vi "comet_thermo_parse_value_html.vi"(8 "error in":errorcluster, 11 "String":string="<!DOCTYPE HTML PUBLIC \"-//W3C//DTD HTML 4.01 Transitional//EN\">\n<html>\n<head>\n <meta http-equiv=\"refresh\" content=\"60\">\n <meta http-equiv=\"content-type\" content=\"text/html; charset=windows-1250\">\n <title>Device: lab7004_JVS</title>\n <style type=\"text/css\">\n <!--\n  h1 {font-size: 1.6em;\tfont-weight: normal;}  \n  .tb {padding:10px 0 0 10px; margin:20px 10px 0 0; height:89px; background:#dee; border:1px solid #000; position:relative;}\n  .ts {padding:0 0 0 0; margin:0 0 0 0; list-style:none; }\n  .ts li {float:left; margin-right:-4px; margin-bottom:-1px;}\n  .ts li a {display:block; text-decoration:none; font-size:11px; font-family:verdana, arial, sans-serif; line-height:23px;}\n  .ts li a em {display:block; float:left; height:25px;text-align:center; padding:0 15px; background:#488; border:1px solid #000; border-right:0; font-style:normal; color:#fff;}\n  .ts li a span {display:none;}\n  .ts li a b {position:relative; display:block; float:left; z-index:100; border-bottom:1px solid #000; width:2px; background:url(tab.gif);}\n  .ts li a b.p1 {height:25px; margin-top:1px;}\n  .ts li a b.p2 {height:23px; margin-top:3px;}\n  .ts li a b.p3 {height:21px; margin-top:5px;}\n  .ts li a b.p4 {height:19px; margin-top:7px;}\n  .ts li a b.p5 {height:18px; width:1px; background:#000; margin-top:9px; font-size:1px; line-height:0; border:0;}\n  .ts li a:hover {color:#000; white-space:normal;}\n  .ts li a:hover em {background:#9bb; color:#000; cursor:pointer; border-bottom-color:#9bb; position:relative; z-index:300;}\n  .ts li a.selected em {background:#9bb; color:#000; border-bottom-color:#9bb; text-decoration:underline; position:relative; z-index:400;}\n  .ts li a.selected:hover em {cursor:default;}\n  .ts li a.selected:hover b {cursor:default;}\n  .ts li a.selected b {z-index:400; background-position:0 -33px; border-bottom-color:#9bb; cursor:pointer;}\n  .ts li a:hover b {background-position:0 -33px; border-bottom-color:#9bb; cursor:pointer;}\n  .ts li a:hover b.p5, .menu li a.selected b.p5 {background:#000;}\n  .ts li a:hover span {display:block; position:absolute; left:10px; top:100px; color:#000; white-space:nowrap;}\n  .ts li a.selected:hover span {display:none;}\n  .info {background:#9bb; border:1px solid #000; border-top:0; padding:12px 10px; margin:0 10px 0px 0; color:#fff; font-size:10px;}\n  .bor {background:#fff; border:1px solid #000; border-top:0; padding:12px 10px; margin:0 10px 0px 0; height:600px;}\n  .lo {background:#99CCFF;}\n  .hi {background:#FFCCCC;}\n  .no {background:#FFFFFF;}\n  .open {background:#FFFFFF;}\n  .closed {background:#FFCCCC;}\n   a:hover { text-decoration:none;}\n   a.tooltip span {display:none; padding:2px 3px; margin-left:8px; white-space:nowrap;}\n   a.tooltip:hover span{display:inline; position:absolute; background:#ffffff; border:1px solid #cccccc; color:#6c6c6c;}\n -->\n </style>\n <link rel=\"alternate\" type=\"application/rss+xml\" title=\"Device: lab7004_JVS values\" href=\"rss1.xml\">\n <link rel=\"alternate\" type=\"application/rss+xml\" title=\"Device: lab7004_JVS alarms\" href=\"rss2.xml\">\n</head>\n\n<body>\n<div class=\"tb\">\n <span style=\"margin-left: 8px;font-size: 2.0em; font-weight: normal;\">Device: lab7004_JVS</span><br>\n <span style=\"margin-left: 8px; font-size: 1.5em; font-weight: normal;\">Serial No: 10963396</span>\n <span style=\"position:absolute; right:10px; top:10px; color:#000;\">Local PC time: <script type=\"text/javascript\">\n<!--\n var d  = new Date();document.write(d.toLocaleString());\n//-->\n</script></span>\n <span style=\"position:absolute; right:10px; top:30px; color:#000;\"><a href=\"http://www.cometsystem.cz\">www.cometsystem.cz</a></span>\n <ul class=\"ts\">\n  <li><a class=\"selected\"><em>Current values</em><b class=\"p1\"></b><b class=\"p2\"></b><b class=\"p3\"></b><b class=\"p4\"></b><b class=\"p5\"></b>\n  </a></li>\n  <li><a href=\"temp.html\"><em>Temperature</em><b class=\"p1\"></b><b class=\"p2\"></b><b class=\"p3\"></b><b class=\"p4\"></b><b class=\"p5\"></b>\n  <span>Temperature history graph.</span></a></li>\n  <li><a href=\"rh.html\"><em>Relative humidity</em><b class=\"p1\"></b><b class=\"p2\"></b><b class=\"p3\"></b><b class=\"p4\"></b><b class=\"p5\"></b>\n  <span>Relative humidity history graph.</span></a></li>\n  <li><a href=\"dp.html\"><em>Dew point</em><b class=\"p1\"></b><b class=\"p2\"></b><b class=\"p3\"></b><b class=\"p4\"></b><b class=\"p5\"></b>\n  <span>Dew point history graph.</span></a></li>\n  <li><a href=\"press.html\"><em>Pressure</em><b class=\"p1\"></b><b class=\"p2\"></b><b class=\"p3\"></b><b class=\"p4\"></b><b class=\"p5\"></b>\n  <span>Pressure history graph.</span></a></li>\n  <li><a href=\"about.html\"><em>About</em><b class=\"p1\"></b><b class=\"p2\"></b><b class=\"p3\"></b><b class=\"p4\"></b><b class=\"p5\"></b>\n  <span>About sensor.</span></a></li>\n  <li><a href=\"tables.html\"><em>Tables >>></em><b class=\"p1\"></b><b class=\"p2\"></b><b class=\"p3\"></b><b class=\"p4\"></b><b class=\"p5\"></b>\n  <span>History tables.</span></a></li>\n </ul>\n</div>\n\n<div class=\"info\"></div>\n<div class=\"bor\">\n <h1>Current measured values:</h1>\n\n <table width=\"530\" border=\"1\" cellpadding=\"5\" cellspacing=\"0\" rules=\"all\">\n  <tr bgcolor=\"#99bbbb\">\n   <td colspan=\"4\" align=\"center\"><b>Analog values</b></td>\n  </tr>\n  <tr bgcolor=\"#ddeeee\">\n   <td><b>Name</b></td>\n   <td colspan=\"2\"><b>Current value</b></td>\n   <td><b>Alarm</b></td>\n  </tr>\n  <tr class=\"no\"> \n   <td>Temperature</td>\n   <td width=\"75\" align=\"right\">22.7</td>\n   <td width=\"75\">°C</td>\n   <td width=\"80\">\n    <a class=\"tooltip\" href=\"temp.html\">no\n    <span>Temperature alarm settings:<br><br>\n    <b>Upper limit:</b>24.5\n    °C<br>\n    <b>Lower limit:</b>21.5\n    °C<br>\n    <b>Hysteresis:</b> 1.0\n    °C<br>\n    <b>Time delay:</b> 120 s</span></a>\n   </td>\n  </tr>\n  <tr class=\"no\">\n   <td>Relative humidity</td>\n   <td align=\"right\">40.3</td>\n   <td>%RH</td>\n   <td>\n    <a class=\"tooltip\" href=\"rh.html\">no\n    <span>Relative humidity alarm settings:<br><br>\n    <b>Upper limit:</b>70.0\n    %RH<br>\n    <b>Lower limit:</b>35.0\n    %RH<br>\n    <b>Hysteresis:</b> 1.0\n    %RH<br>\n    <b>Time delay:</b> 120 s</span></a>\n   </td> \n  </tr>\n  <tr class=\"no\">\n   <td>Dew point</td>\n   <td align=\"right\">8.5</td>\n   <td>°C</td>\n   <td>\n    <a class=\"tooltip\" href=\"dp.html\">no\n    <span>Dew point alarm settings:<br><br>\n    <b>Upper limit:</b>80.0\n    °C<br>\n    <b>Lower limit:</b>-50.0\n    °C<br>\n    <b>Hysteresis:</b> 1.0\n    °C<br>\n    <b>Time delay:</b> 120 s</span></a>\n   </td>\n  </tr>\n  <tr class=\"no\">\n   <td>Pressure</td>\n   <td align=\"right\">987.0</td>\n   <td>hPa</td>\n   <td>\n    <a class=\"tooltip\" href=\"press.html\">no\n    <span>Pressure alarm settings:<br><br>\n    <b>Upper limit:</b>1100.0\n    hPa<br>\n    <b>Lower limit:</b>600.0\n    hPa<br>\n    <b>Hysteresis:</b> 1.0\n    hPa<br>\n    <b>Time delay:</b> 120 s</span></a>\n   </td>  \n  </tr>\n </table>\n\n <br>\n\n</div>\n<!--WZ-REKLAMA-1.0IZ--><script type='text/javascript'><!--//<![CDATA[\n   var m3_u = (location.protocol=='https:'?'https':'http')+'://ad.wz.cz/openx/www/delivery/ajs.php';\n   var m3_r = Math.floor(Math.random()*99999999999);\n   if (!document.MAX_used) document.MAX_used = ',';\n   document.write (\"<scr\"+\"ipt type='text/javascript' src='\"+m3_u);\n   document.write (\"?zoneid=44\");\n   document.write ('&amp;cb=' + m3_r);\n   if (document.MAX_used != ',') document.write (\"&amp;exclude=\" + document.MAX_used);\n   document.write (document.charset ? '&amp;charset='+document.charset : (document.characterSet ? '&amp;charset='+document.characterSet : ''));\n   document.write (\"&amp;loc=\" + escape(window.location));\n   if (document.referrer) document.write (\"&amp;referer=\" + escape(document.referrer));\n   if (document.context) document.write (\"&context=\" + escape(document.context));\n   if (document.mmm_fo) document.write (\"&amp;mmm_fo=1\");\n   document.write (\"'><\\/scr\"+\"ipt>\");\n//]]>--></script><noscript><div><a href='http://ad.wz.cz/openx/www/delivery/ck.php?n=a5977468&amp;cb=123'><img src='http://ad.wz.cz/openx/www/delivery/avw.php?zoneid=44&amp;cb=123&amp;n=a5977468' style='margin: 0; padding: 0; border-width: 0' alt='' /></a></div></noscript>\n<!--WZ-REKLAMA-1.0IK--></body>\n</html>\n") -> (0 "error out":errorcluster, 1 "p [hPa]":dbl, 2 "RH [%]":dbl, 3 "t [C]":dbl, 5 "p4":dbl)   [LabVIEW 2020]
uses:
  <vilib>/regexp/Match Regular Expression.xnode
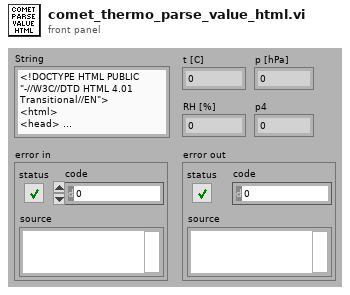
[diagram p1: front panel]
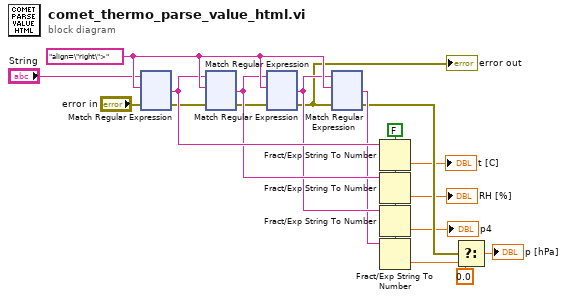
[diagram p0: block diagram]
diagram:
  w13 = FALSE ("use system decimal point (T)")
  w18 = "align=\"right\">" ("regular expression")
  n1 = xnode "Match Regular Expression"("input string"="String", "regular expression"=w18, "error in"="error in") -> ("after match"=w17:string, "error out"=w9:errorcluster)  [unwired: 3 in, 3 out]
  n2 = xnode "Match Regular Expression"("input string"=w17, "regular expression"=w18, "error in"=w9) -> ("after match"=w16:string, "error out"=w10:errorcluster)  [unwired: 3 in, 3 out]
  n3 = xnode "Match Regular Expression"("input string"=w16, "regular expression"=w18, "error in"=w10) -> ("after match"=w15:string, "error out"=w11:errorcluster)  [unwired: 3 in, 3 out]
  "error out" <- w11
  n4 = xnode "Match Regular Expression"("input string"=w15, "regular expression"=w18, "error in"=w11) -> ("after match"=w14:string, "error out"=w12:errorcluster)  [unwired: 3 in, 3 out]
  n5 = Fract/Exp String To Number(use system decimal point (T)=w13, string=w17) -> (number=→"t [C]":dbl)  [unwired: 2 in, 1 out]
  n6 = Fract/Exp String To Number(use system decimal point (T)=w13, string=w16) -> (number=→"RH [%]":dbl)  [unwired: 2 in, 1 out]
  n7 = Fract/Exp String To Number(use system decimal point (T)=w13, string=w15) -> (number=→"p4":dbl)  [unwired: 2 in, 1 out]
  n8 = Fract/Exp String To Number(use system decimal point (T)=w13, string=w14) -> (number=w8:dbl)  [unwired: 2 in, 1 out]
  n9 = Select(t=0.0, s=w12, f=w8) -> (s? t:f=→"p [hPa]":dbl)
